vi "PH_BeamlineController.PC Set-Target.vi"(0 "i ref in":refnum<vi>, 2 "Targets":T1, 3 "Value":bool, 5 "error in (no error)":errorcluster) -> (14 "i ref out":refnum<vi>, 17 "Targets changed?":bool, 19 "error out":errorcluster)   [LabVIEW 2014, in "PH_BeamlineController.lvlib"]
doc: "This VI writes incoming Information to own Attributes if the new value differs from the stored."
uses:
  PH_BeamlineController.lvlib
  PH_BeamlineController.Targets.ctl
  PH_SystemInformation/PH_SystemInformationEnabling State.ctl
  PH_BeamlineController.PA DP Targets.ctl
  PH_SystemInformation/PH_SystemInformation.lvlib
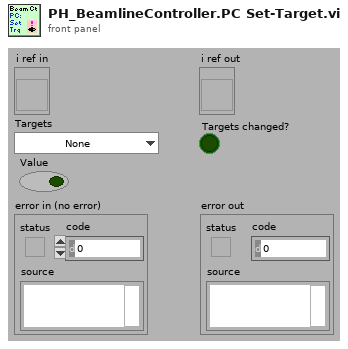
[diagram p1: front panel]
types:
  T1 = typedef "PH_BeamlineController.lvlib/PH_BeamlineController.Targets.ctl" = enum16{"None", "PreAmp", "Dump Exp Laserlab", "Exp Laserlab", "Calorimeter", "Dump Exp Laserbay", "Exp Laserbay", "Dump Exp Z6", "Exp Z6"}
  T2 = enum16{"Laser", "PreAmp", "MainAmp", "Exp 1", "Exp 2", "Exp 3", "Exp 4"}
  T3 = typedef "PH_SystemInformation.lvlib/PH_SystemInformationEnabling State.ctl" = i32
  T4 = typedef "PH_BeamlineController.lvlib/PH_BeamlineController.PA DP Targets.ctl" = enum16{"None", "Dump PA Delayed Beam", "Dump PA Undelayed Beam", "Dumps PA Delayed and Undelayed Beam"}
  T5 = typedef "PH_BeamlineController.lvlib/PH_BeamlineController.Target Attributes.ctl" = cluster{"Name":T1, "GUI Ref":refnum<vi>, "Current State":bool, "Wanted State":bool, "Enabled":bool}
  T6 = typedef "PH_BeamlineController.lvlib/PH_BeamlineController.i attribute.ctl" = cluster{"Vacuum Exp LB":cluster{"Channel":string, "Limit [mbar]":dbl, "Pressure [mbar]":dbl, "GUI Ref":refnum<vi>}, "Sources":T7[], "PA DP Targets":T9[], "Path":cluster{"Source":T8, "PA DP Target":T4, "Target":T1}, "Targets":cluster{"Name":T1, "GUI Ref":refnum<vi>, "Current State":bool, "Wanted State":bool, "Enabled":bool}[], "Status Tags":cluster{"Name":string, "Status":T10}[], "special GUI Refs":T11}
  T7 = typedef "PH_BeamlineController.lvlib/PH_BeamlineController.Source Attributes.ctl" = cluster{"Name":T8, "GUI Ref":refnum<vi>, "Current State":bool, "Wanted State":bool}
  T8 = typedef "PH_BeamlineController.lvlib/PH_BeamlineController.Sources.ctl" = enum16{"None", "YLF", "fs-Frontend", "ns-Frontend", "YLF and ns-Frontend", "fs- and ns-Frontend"}
  T9 = typedef "PH_BeamlineController.lvlib/PH_BeamlineController.PA DP Target Attributes.ctl" = cluster{"Name":T4, "GUI Ref":refnum<vi>, "Current State":bool, "Wanted State":bool, "Enabled":bool}
  T10 = typedef "PH_StatusHandler.lvlib/PH_StatusHandler.Status.ctl" = i16
  T11 = typedef "PH_BeamlineController.lvlib/PH_BeamlineController.special GUI Refs.ctl" = cluster{"PA-Backreflection-Meas":refnum<vi>, "fs_Synchrolock_Watch":refnum<vi>}
  T12 = cluster{"Name":T1, "GUI Ref":refnum<vi>, "Current State":bool, "Wanted State":bool, "Enabled":bool}[]
  T13 = cluster{"Name":T1, "GUI Ref":refnum<vi>, "Current State":bool, "Wanted State":bool, "Enabled":bool}
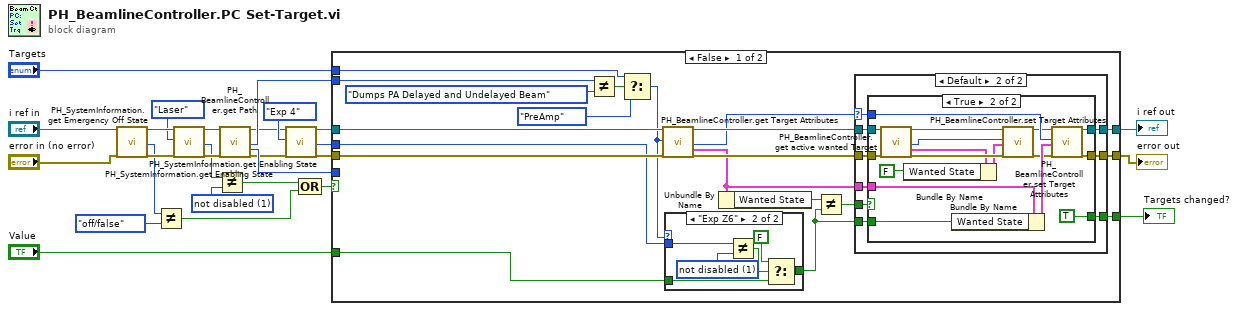
[diagram p0: block diagram]
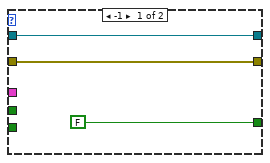
[diagram p3: hidden frame]
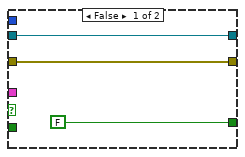
[diagram p4: hidden frame]
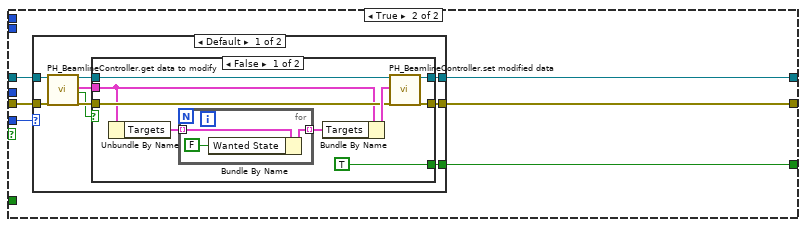
[diagram p5: hidden frame]
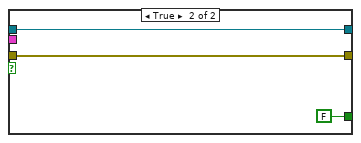
[diagram p6: hidden frame]
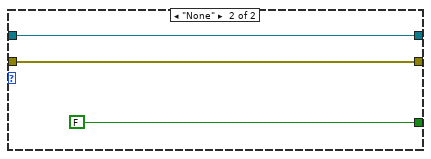
[diagram p7: hidden frame]
diagram:
  w14 = T3 1 items=["no info", "not disabled", "disabled"] ("y")
  n1 = call "PH_SystemInformation.get Emergency Off State.vi"("i ref in"="i ref in", "error in (no error)"="error in (no error)") -> ("i ref out"=w23:refnum<vi>, "Emergency Off State"=w13:enum16{"no info", "off/false", "Alarm"}, "error out"=w22:errorcluster)  [unwired: 15 in]
  n2 = Not Equal?(x=w13, y=enum16{"no info", "off/false", "Alarm"}."off/false") -> (x != y?=w10:bool)
  n3 = call "PH_SystemInformation.get Enabling State.vi"("i ref in"=w23, "Wanted State"=T2."Laser", "error in (no error)"=w22) -> ("i ref out"=w17:refnum<vi>, "Enabling State"=w12:T3, "error out"=w16:errorcluster)  [unwired: 14 in]
  n4 = Not Equal?(x=w12, y=w14) -> (x != y?=w11:bool)
  n5 = call "PH_BeamlineController.get Path.vi"("VI in"=w17, "error in (no error)"=w16) -> ("VI out"=w2:refnum<vi>, "Path:  PA DP Targets"=w3:T4, "Path: Target"=w4:T1, "error out"=w1:errorcluster)  [unwired: 12 in, 2 out]
  n6 = call "PH_SystemInformation.get Enabling State.vi"("i ref in"=w2, "Wanted State"=T2."Exp 4", "error in (no error)"=w1) -> ("i ref out"=w7:refnum<vi>, "Enabling State"=w5:T3, "error out"=w8:errorcluster)  [unwired: 14 in]
  n7 = Compound Arithmetic op=OR(w11, w10) -> (w9:bool)
  n8 = case shown="False" w9 {
    tunnel: [w47 w88] -> w27
    tunnel: [w46 w89] -> w26
    tunnel: "Targets" -> [w30 _]
    tunnel: [w45 w87] -> w24
    tunnel: "Value" -> [w36 _]
    tunnel: w7 -> [w38 w90]
    tunnel: w8 -> [w37 w91]
    tunnel: w4 -> [_ w92]
    tunnel: w5 -> [w34 _]
    tunnel: w3 -> [w33 _]
    frame False {
      n9 = Not Equal?(x=w33, y=PH_BeamlineController.PA_DP_Targets."Dumps PA Delayed and Undelayed Beam") -> (x != y?=w31:bool)
      n10 = Select(t=w30, s=w31, f=PH_BeamlineController.Targets."PreAmp") -> (s? t:f=w29:T1)
      n11 = call "PH_BeamlineController.get Target Attributes.vi"("VI in"=w38, "Target"=w29, "error in (no error)"=w37) -> ("VI out"=w43:refnum<vi>, "Target Index"=w39:i32, "Target Attributes"=w42:T5, "error out"=w44:errorcluster)  [unwired: 13 in]
      n12 = case shown="\"Exp Z6\"" w29 {
        tunnel: w36 -> [w48 w53]
        tunnel: [w48 w52] -> w35
        tunnel: w34 -> [_ w50]
        frame Default {
        }
        frame "Exp Z6" {
          w49 = T3 1 items=["no info", "not disabled", "disabled"] ("Enabling State")
          n13 = Not Equal?(x=w50, y=w49) -> (x != y?=w54:bool)
          n14 = Select(t=FALSE, s=w54, f=w53) -> (s? t:f=w52:bool)
        }
      }
      n15 = Unbundle By Name(w42) -> ("Wanted State"=w41:bool)
      n16 = Not Equal?(x=w41, y=w35) -> (x != y?=w40:bool)
      n17 = case shown="Default" w39 {
        selector: w39 -> [_ w58]
        tunnel: [w56 w66] -> w47
        tunnel: [w57 w65] -> w46
        tunnel: w44 -> [w56 w64]
        tunnel: w43 -> [w57 w63]
        tunnel: w35 -> [_ w62]
        tunnel: w42 -> [_ w61]
        tunnel: w40 -> [_ w60]
        tunnel: [FALSE w59] -> w45
        frame -1 {
        }
        frame Default {
          n18 = case shown="True" w60 {
            tunnel: [w69 w80] -> w65
            tunnel: [w68 w79] -> w66
            tunnel: w64 -> [w68 w86]
            tunnel: w63 -> [w69 w78]
            tunnel: w58 -> [_ w85]
            tunnel: w61 -> [_ w84]
            tunnel: w62 -> [_ w82]
            tunnel: [FALSE TRUE] -> w59
            frame False {
            }
            frame True {
              n19 = call "PH_BeamlineController.get active wanted Target.vi"("VI in"=w78, "error in (no error)"=w86) -> ("VI out"=w77:refnum<vi>, "active wanted State Index"=w73:i32, "active wanted State Target Attributes"=w72:T5, "error out"=w75:errorcluster)  [unwired: 14 in]
              n20 = Bundle By Name(cluster=w72, "Wanted State"=FALSE) -> (w71:T5)
              n21 = Bundle By Name(cluster=w84, "Wanted State"=w82) -> (w83:T5)
              n22 = call "PH_BeamlineController.set Target Attributes.vi"("VI in"=w77, "Target Index"=w73, "Changed Target Attributes"=w71, "error in (no error)"=w75) -> ("VI out"=w76:refnum<vi>, "error out"=w74:errorcluster)  [unwired: 14 in]
              n23 = call "PH_BeamlineController.set Target Attributes.vi"("VI in"=w76, "Target Index"=w85, "Changed Target Attributes"=w83, "error in (no error)"=w74) -> ("VI out"=w80:refnum<vi>, "error out"=w79:errorcluster)  [unwired: 14 in]
            }
          }
        }
      }
    }
    frame True {
      n24 = case shown="Default" w92 {
        tunnel: w91 -> [w96 w118]
        tunnel: w90 -> [w97 w119]
        tunnel: [w95 w119] -> w89
        tunnel: [w94 w118] -> w88
        tunnel: [w93 FALSE] -> w87
        frame Default {
          n25 = call "PH_BeamlineController.get data to modify.vi"("i ref in"=w97, "error in (no error)"=w96) -> ("i ref out"=w101:refnum<vi>, "i attribute"=w99:T6, "timed out"=w98:bool, "error out"=w100:errorcluster)  [unwired: 14 in]
          n26 = case shown="False" w98 {
            tunnel: w101 -> [w107 w116]
            tunnel: [w110 w116] -> w95
            tunnel: w100 -> [w106 w115]
            tunnel: [w109 w115] -> w94
            tunnel: w99 -> [w105 _]
            tunnel: [TRUE FALSE] -> w93
            frame False {
              n27 = Unbundle By Name(w105) -> ("Targets"=w104:T12)
              n28 = for {
                tunnel: w104 -> [w113] mode=indexing
                tunnel: [w112] -> w103 mode=indexing
                n29 = Bundle By Name(cluster=w113, "Wanted State"=FALSE) -> (w112:T13)
              }
              n30 = Bundle By Name(cluster=w105, "Targets"=w103) -> (w108:T6)
              n31 = call "PH_BeamlineController.set modified data.vi"("i ref in"=w107, "i attribute"=w108, "error in (no error)"=w106) -> ("i ref out"=w110:refnum<vi>, "error out"=w109:errorcluster)  [unwired: 15 in]
            }
            frame True {
            }
          }
        }
        frame "None" {
        }
      }
    }
  }
  "error out" <- w27
  "i ref out" <- w26
  "Targets changed?" <- w24
